vi "AliasingCorr9225-7_FPGA.vi"(0 "iMAX":u16, 1 "Real{a}":fxp<+/-,36,0>, 2 "Imag{a}":fxp<+/-,36,0>, 5 "dBin":fxp<+/-,36,0>, 7 "Amplitude":fxp<+,36,0>, 9 "phase(floor(iMAX+dBin))":fxp<+/-,36,2>, 11 "Dbin<0":bool, 12 "Real{b}":fxp<+/-,36,0>, 13 "Imag{b}":fxp<+/-,36,0>) -> (4 "AA(a) [p.u.]":fxp<+,36,0>, 8 "AA(b) [p.u.]":fxp<+,36,0>, 15 "AA(phase(a)) [pi]":fxp<+/-,36,2>)   [LabVIEW 2021]
uses:
  <vilib>/rvi/FXPMathLib/FxpAdd/XNode/nifxpmath_Add.xnode
  <vilib>/rvi/FXPMathLib/FxpSub/XNode/nifxpmath_Sub.xnode
  <vilib>/rvi/FXPMathLib/sim/FxpSim.dll
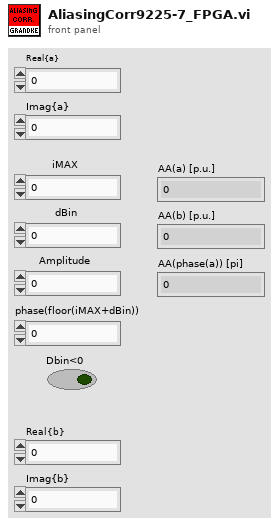
[diagram p1: front panel]
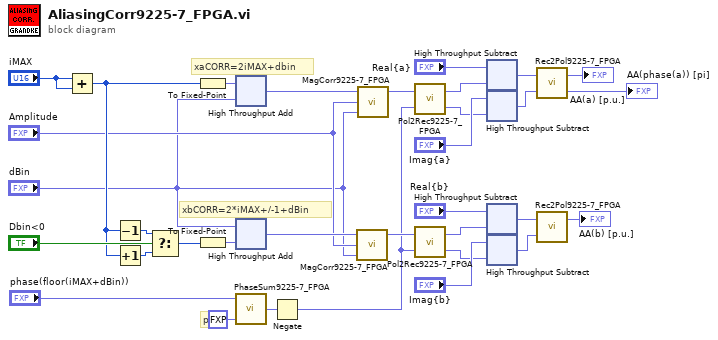
[diagram p0: block diagram]
diagram:
  # "xaCORR=2iMAX+dbin"
  # "xbCORR=2*iMAX+/-1+dBin"
  # "pi"
  n1 = Add(x="iMAX", y="iMAX") -> (x+y=w23:u16)
  n2 = Decrement(x=w23) -> (x-1=w33:u16)
  n3 = Increment(x=w23) -> (x+1=w32:u16)
  n4 = Select(t=w33, s="Dbin<0", f=w32) -> (s? t:f=w22:u16)
  n5 = To Fixed-Point(number=w23) -> (fixed-point=w30:fxp<+,16,16>)  [unwired: 1 in]
  n6 = To Fixed-Point(number=w22) -> (fixed-point=w31:fxp<+,16,16>)  [unwired: 1 in]
  n7 = xnode "High Throughput Add"("x"=w30, "y"="dBin") -> ("x+y"=w4:fxp<+,36,4>)
  n8 = xnode "High Throughput Add"("x"="dBin", "y"=w31) -> ("x+y"=w3:fxp<+,36,4>)
  n9 = call "PhaseSum9225-7_FPGA.vi"("phi2 [pi rad]"=fxp<+/-,36,2> 1.0 ("x"), "phi1 [pi rad]"="phase(floor(iMAX+dBin))") -> ("phi1+phi2 [pi rad] (-1,1]"=w25:fxp<+/-,36,2>)  [unwired: 3 in]
  n10 = Negate(x=w25) -> (-x=w14:fxp<+/-,36,2>)
  n11 = call "MagCorr9225-7_FPGA.vi"("dBin"="dBin", "A"="Amplitude", "xCORR"=w3) -> ("rCORR"=w15:fxp<+,36,0>)  [unwired: 2 in]
  n12 = call "MagCorr9225-7_FPGA.vi"("dBin"="dBin", "A"="Amplitude", "xCORR"=w4) -> ("rCORR"=w18:fxp<+,36,0>)  [unwired: 2 in]
  n13 = call "Pol2Rec9225-7_FPGA.vi"("phase [pi]"=w14, "magnitude"=w18) -> ("Im"=w16:fxp<+/-,36,0>, "Re"=w17:fxp<+/-,36,0>)
  n14 = call "Pol2Rec9225-7_FPGA.vi"("phase [pi]"=w14, "magnitude"=w15) -> ("Im"=w12:fxp<+/-,36,0>, "Re"=w13:fxp<+/-,36,0>)
  n15 = xnode "High Throughput Subtract"("x"="Real{a}", "y"=w17) -> ("x-y"=w9:fxp<+/-,36,0>)
  n16 = xnode "High Throughput Subtract"("x"="Imag{a}", "y"=w16) -> ("x-y"=w8:fxp<+/-,36,0>)
  n17 = xnode "High Throughput Subtract"("x"="Real{b}", "y"=w13) -> ("x-y"=w6:fxp<+/-,36,0>)
  n18 = xnode "High Throughput Subtract"("x"="Imag{b}", "y"=w12) -> ("x-y"=w5:fxp<+/-,36,0>)
  n19 = call "Rec2Pol9225-7_FPGA.vi"("Imag"=w8, "Real"=w9) -> ("phase [pi]"=→"AA(phase(a)) [pi]":fxp<+/-,36,2>, "magnitude [p.u.]"=→"AA(a) [p.u.]":fxp<+,36,0>)
  n20 = call "Rec2Pol9225-7_FPGA.vi"("Imag"=w5, "Real"=w6) -> ("magnitude [p.u.]"=→"AA(b) [p.u.]":fxp<+,36,0>)  [unwired: 1 out]
